vi "call.vi"   [LabVIEW 2017]
uses:
  resource/dialog/QuickDrop/plugins/QD_String to Enum/String to Enum.lvlib
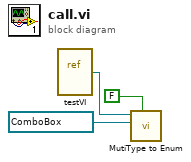
[diagram p0: block diagram]
diagram:
  n1 = vi-ref "testVI.vi"() -> (w1:refnum<vi>)
  n2 = call "MutiType to Enum.vi"("Shift Pressed?"=FALSE, "QD Combo Box Ref"=refnum<vi> refnum, "QD Launch VI Ref"=w1) -> ()  [unwired: 7 in, 2 out]
